vi "MDAQ_FileParser.vi"(8 "error in":errorcluster, 11 "ReadData":string) -> (0 "error out":errorcluster, 1 "Raw Data":string[](array[string]), 2 "Run Info":T1)   [LabVIEW 2021]
uses:
  XML_Cluster.ctl
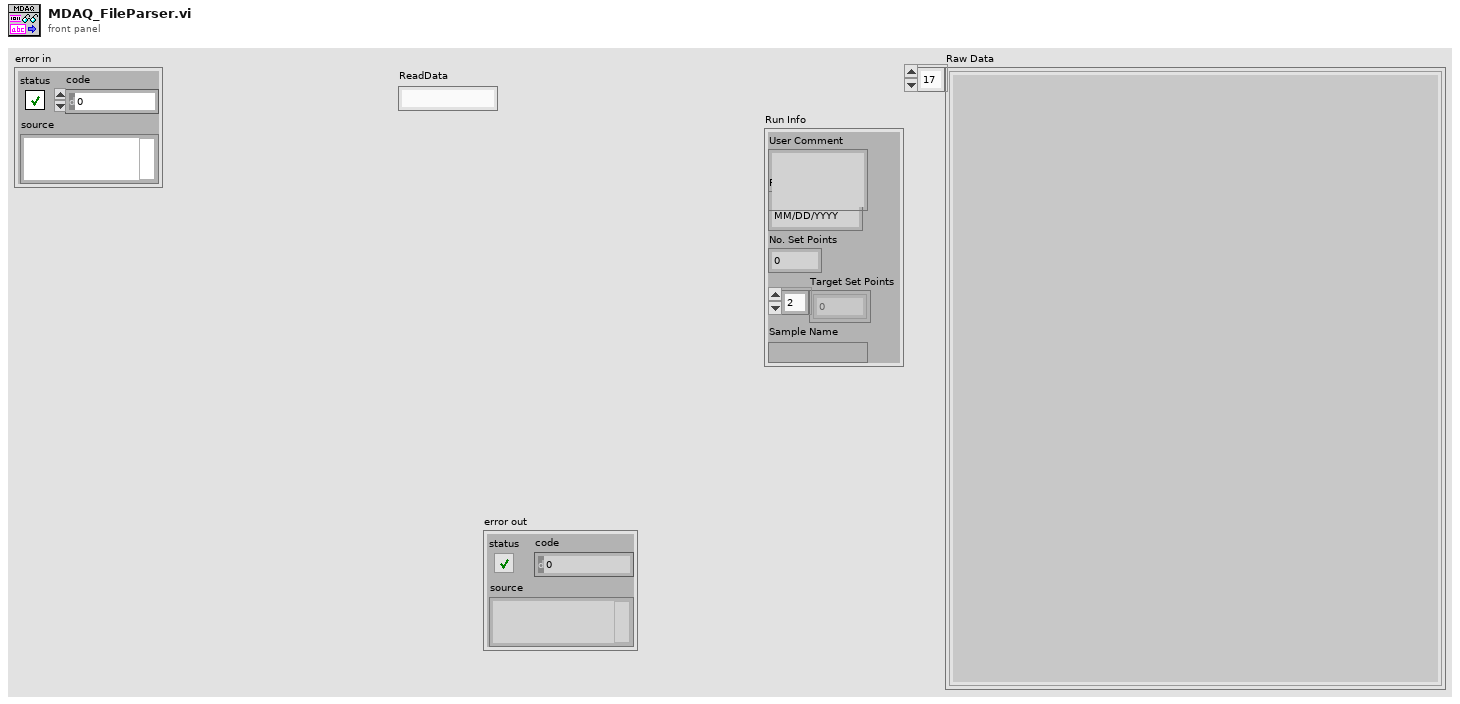
[diagram p1: front panel]
types:
  T1 = typedef "XML_Cluster.ctl" = cluster{"User Comment":string, "Run Start TimeS":timestamp, "No. Set Points":u32, "Target Set Points":i32[], "Sample Name":string}
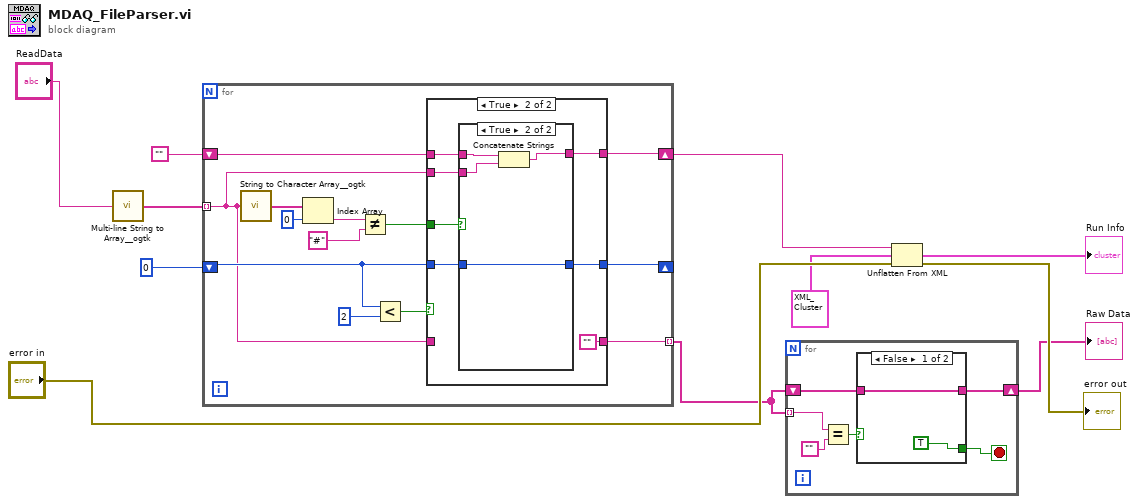
[diagram p0: block diagram]
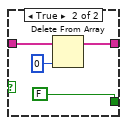
[diagram p2: hidden frame]
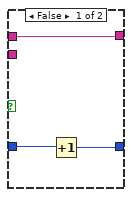
[diagram p4: hidden frame]
diagram:
  n1 = call <userlib>:"Multi-line String to Array__ogtk.vi"("string"="ReadData") -> ("lines"=w10:string[])
  n2 = for {
    tunnel: w10 -> [w12] mode=indexing
    shift-right: [w19] -> w7
    shift-left: "" -> [w18]
    shift-right: [w17] -> _
    shift-left: 0 -> [w16]
    tunnel: [w13] -> w2 mode=indexing
    n3 = call <userlib>:"String to Character Array__ogtk.vi"("Input String"=w12) -> ("Character Array"=w24:string[])
    n4 = Index Array(array=w24, index=0) -> (element=w22:string)
    n5 = Not Equal?(x=w22, y="#") -> (x != y?=w20:bool)
    n6 = Less?(x=w16, y=2) -> (x < y?=w14:bool)
    n7 = case shown="True" w14 {
      tunnel: w20 -> [_ w34]
      tunnel: w12 -> [_ w33]
      tunnel: [w26 w32] -> w19
      tunnel: w18 -> [w26 w31]
      tunnel: [w25 w30] -> w17
      tunnel: w16 -> [w25 w29]
      tunnel: [w27 ""] -> w13
      tunnel: w12 -> [w27 _]
      frame False {
      }
      frame True {
        n8 = case shown="True" w34 {
          tunnel: w33 -> [_ w39]
          tunnel: [w37 w41] -> w32
          tunnel: w31 -> [w37 w40]
          tunnel: [w36 w38] -> w30
          tunnel: w29 -> [w35 w38]
          frame False {
            n9 = Increment(x=w35) -> (x+1=w36:i32)
          }
          frame True {
            n10 = Concatenate Strings(w40, w39) -> (w41:string)
          }
        }
      }
    }
  }
  n11 = for {
    tunnel: w2 -> [w45] mode=indexing
    shift-right: [w43] -> w1
    shift-left: w2 -> [w47]
    stop <- w42 stop-if-true
    n12 = Equal?(x=w45, y="") -> (x = y?=w44:bool)
    n13 = case shown="False" w44 {
      tunnel: w47 -> [w49 w51]
      tunnel: [w49 w53] -> w43
      tunnel: [TRUE FALSE] -> w42
      frame False {
      }
      frame True {
        n14 = Delete From Array(array=w51, index=0) -> (array with subset deleted=w53:string[])  [unwired: 1 in, 1 out]
      }
    }
  }
  "Raw Data" <- w1
  n15 = Unflatten From XML(xml string=w7, type=T1 {"User Comment"="", "Run Start TimeS"=timestamp(0 s since 1904-01-01), "No. Set Points"=0, "Target Set Points"=[], "Sample Name"=""} ("Cluster"), error in (no error)="error in") -> (value=→"Run Info":T1, error out=→"error out":errorcluster)
